vi "motor safety.vi"(0 "Desired Rate":dbl, 1 "Encoder Refnum":string="turret", 5 "Forward Limit":dbl, 9 "Reverse Limit":dbl, 11 "Cutoff Rate":dbl=0.2, 12 "Max Rate":dbl=50.0, 13 "Min Rate":dbl) -> (3 "Limit":bool, 8 "Rate Output":dbl, 14 "Cutoff Tripped":bool)   [LabVIEW 2013]
doc: "This VI provides two types of safety for your motors. An encoder for the motor is required. If the encoder reference is innalid, the motor won't be allowed to run. \nThe first safetyis a distance limit. The forward and reverse limit parameters specify the max and min valus for the encoder distance to read until the motor is stopped and only allowed to move away from its limit. \nThe second safety is an encoder safety. The Cutoff Rate parameter is the maximum value allowed to be sent to the motor without a response seen from the encoder. So, if the code is trying to set a value higher than this parameter and the encoder doesn't register a response, the motor will be disabled. It will be reenabled when movement is registered from the encoder. This safety will also permanately disable the motor if the encoder reads some inanely high rate. Consider a replacement...."
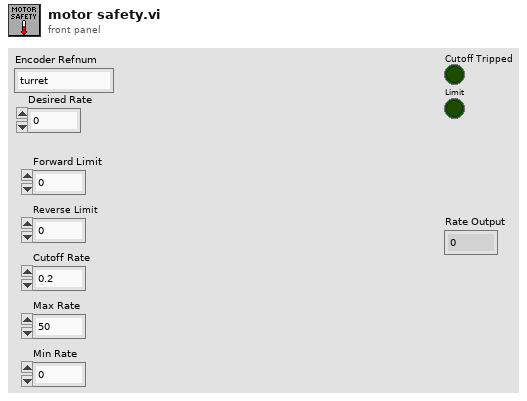
[diagram p1: front panel]
types:
  T1 = typedef "WPI_EncoderDevRef.ctl" = cluster{"DevStatus":errorcluster, "EncoderIndex":T2, "CounterIndex":T3, "DistancePerCount":dbl, "Decoding Type":T4}
  T2 = typedef "FPGA_EncoderIdx.ctl" = enum8{"Enc 0", "Enc 1", "Enc 2", "Enc 3", "Invalid"}
  T3 = typedef "FPGA_CounterCtrSystemIndex.ctl" = enum8{"Ctr 0", "Ctr 1", "Ctr 2", "Ctr 3", "Ctr 4", "Ctr 5", "Ctr 6", "Ctr 7", "Invalid"}
  T4 = typedef "WPI_EncoderType.ctl" = enum16{"1x", "2x", "4x"}
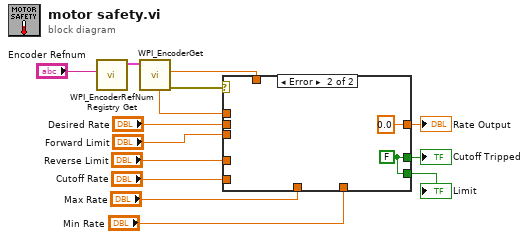
[diagram p0: block diagram]
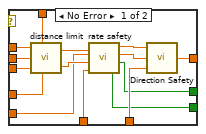
[diagram p2: hidden frame]
diagram:
  n1 = call <vilib>:"WPI_EncoderRefNum Registry Get.vi"("refnum name"="Encoder Refnum") -> ("EncoderDevRef"=w13:T1)  [unwired: 9 in, 1 out]
  n2 = call <vilib>:"WPI_EncoderGet.vi"("EncoderDevRef"=w13) -> ("error out"=w5:errorcluster, "Distance"=w10:dbl, "Rate"=w12:dbl)  [unwired: 5 in, 3 out]
  n3 = case shown="Error" w5 {
    tunnel: w12 -> [w29 _]
    tunnel: "Desired Rate" -> [w28 _]
    tunnel: w10 -> [w25 _]
    tunnel: [w17 0.0 ("Output Rate")] -> w9
    tunnel: "Forward Limit" -> [w24 _]
    tunnel: "Reverse Limit" -> [w23 _]
    tunnel: "Cutoff Rate" -> [w22 _]
    tunnel: "Max Rate" -> [w21 _]
    tunnel: "Min Rate" -> [w18 _]
    tunnel: [w16 w30] -> w2
    tunnel: [w15 w30] -> w1
    frame No Error {
      n4 = call "distance limit.vi"("Encoder Rate"=w29, "Encoder Distance"=w25, "Desired Rate"=w28, "Forward Limit"=w24, "Reverse Limit"=w23) -> ("Encoder Rate Out"=w27:dbl, "Output Rate"=w26:dbl)
      n5 = call "rate safety.vi"("Max Rate"=w21, "Desired Rate"=w26, "Cutoff Rate"=w22, "Encoder Rate"=w27) -> ("Limit"=w15:bool, "Cutoff Tripped"=w16:bool, "Output Rate"=w19:dbl, "Encoder Rate Out"=w20:dbl)
      n6 = call "Direction Safety.vi"("Min Rate"=w18, "Desired Rate"=w19, "Encoder Rate"=w20) -> ("Super Safe Rate"=w17:dbl)
    }
    frame Error {
      w30 = FALSE ("Cutoff Tripped")
    }
  }
  "Rate Output" <- w9
  "Cutoff Tripped" <- w2
  "Limit" <- w1
